vi "BK Precision 983X Series Create List Program.vi"() -> ()   [LabVIEW 2015]
doc: "This example demonstrates how to create a simple list program and stored into internal memory."
uses:
  <instrlib>/BK Precision 983X Series/BK Precision 983X Series.lvlib
panel:
  in  "List Step Voltage":T1 {"End DC Voltage (0 V)" format="%.3g"; "End AC Voltage (0 V)" format="%.3g"; "Start DC Voltage (0 V)" format="%.3g"; "Start AC Voltage (0 V)" format="%.3g"}
  in  "End Frequency (50 Hz)":dbl=50.0 min=43.0 max=1200.0 format="%.3g"
  in  "Start Frequency (50 Hz)":dbl=50.0 min=43.0 max=1200.0 format="%.3g"
  in  "List Step Time Cycle (1 ms/cycles)":u32=1 min=1 max=100000
  in  "List Step Count (0)":u32 max=200 step=1
  in  "Enable Infinite Mode (F: False)":bool
  in  "List Timing Mode (0:Time)":i32(ring) items=["Time", "Cycle"]
  in  "List Phase (0.0 degrees)":dbl min=0.0 max=359.7 format="%.1g"
  in  "List Sync (0: Immediate)":i32(ring) items=["Immediate", "Phase"]
  in  "Repeat Count (0)":u32 max=99 step=1
  in  "VISA resource name":refnum<visa-resource-name>
  # "(c) 2017 B&K Precision Corporation.  ALL RIGHTS RESERVED."
  # "V"
  # "V"
  # "V"
  # "V"
  # "Hz"
  # "Hz"
  # "degree"
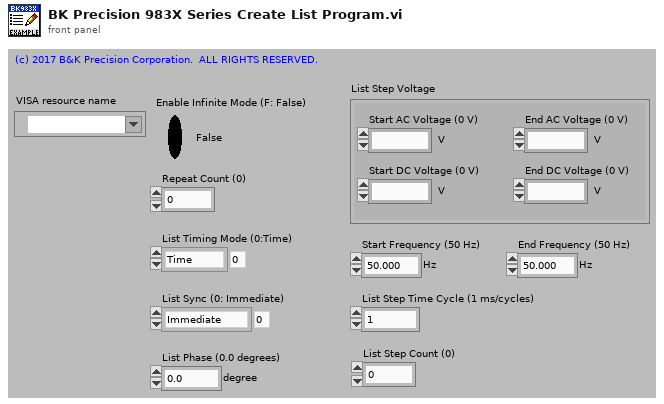
[diagram p1: front panel]
types:
  T1 = cluster{"Start AC Voltage (0 V)":dbl, "Start DC Voltage (0 V)":dbl, "End AC Voltage (0 V)":dbl, "End DC Voltage (0 V)":dbl}
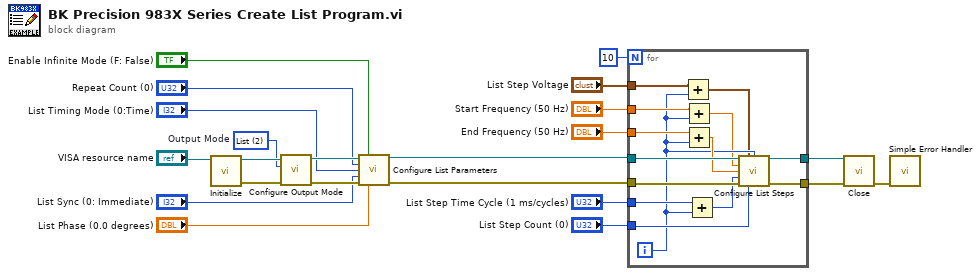
[diagram p0: block diagram]
diagram:
  w16 = u16 2 items=["Normal", "Step", "List", "Pulse"]  # Output Mode
  n1 = call <instrlib>:"Initialize.vi"("VISA resource name"="VISA resource name") -> ("error out"=w19:errorcluster, "VISA resource name out"=w20:refnum<visa-resource-name>)  [unwired: 9 in]
  n2 = call <instrlib>:"Configure Output Mode.vi"("error in (no error)"=w19, "Output Mode (0:Normal)"=w16, "VISA resource name"=w20) -> ("error out"=w17:errorcluster, "VISA resource name out"=w18:refnum<visa-resource-name>)  [unwired: 7 in]
  n3 = call <instrlib>:"Configure List Parameters.vi"("VISA resource name"=w18, "Enable Infinite Mode (F: False)"="Enable Infinite Mode (F: False)", "Repeat Count (0)"="Repeat Count (0)", "List Timing Mode (0:Time)"="List Timing Mode (0:Time)", "List Sync (0: Immediate)"="List Sync (0: Immediate)", "error in (no error)"=w17, "List Phase (0.0 degrees)"="List Phase (0.0 degrees)") -> ("VISA resource name out"=w10:refnum<visa-resource-name>, "error out"=w9:errorcluster)  [unwired: 7 in]
  n4 = for {
    N: 10 -> [_]
    tunnel: w10 -> [w36]
    tunnel: w9 -> [w35]
    tunnel: "List Step Voltage" -> [w26]
    tunnel: "Start Frequency (50 Hz)" -> [w27]
    tunnel: "End Frequency (50 Hz)" -> [w28]
    tunnel: "List Step Time Cycle (1 ms/cycles)" -> [w31]
    tunnel: "List Step Count (0)" -> [w32]
    tunnel: [w34] -> w2
    tunnel: [w33] -> w1
    i -> [w25]
    n5 = Add(x=w26, y=w25) -> (x+y=w23:T1)
    n6 = Add(x=w27, y=w25) -> (x+y=w24:dbl)
    n7 = Add(x=w28, y=w25) -> (x+y=w29:dbl)
    n8 = Add(x=w31, y=w25) -> (x+y=w30:u32)
    n9 = call <instrlib>:"Configure List Steps.vi"("VISA resource name"=w36, "List Step Voltage"=w23, "Step Number (0)"=w25, "Start Frequency (50 Hz)"=w24, "End Frequency (50 Hz)"=w29, "List Step Time Cycle (1 ms/cycles)"=w30, "error in (no error)"=w35, "List Step Count (0)"=w32) -> ("VISA resource name out"=w34:refnum<visa-resource-name>, "error out"=w33:errorcluster)  [unwired: 6 in]
  }
  n10 = call <instrlib>:"Close.vi"("error in (no error)"=w1, "VISA resource name"=w2) -> ("error out"=w21:errorcluster)  [unwired: 9 in]
  n11 = call <vilib>:"Simple Error Handler.vi"("error in (no error)"=w21) -> ()  [unwired: 4 in, 5 out]
